vi "test.vi"() -> ()   [LabVIEW 2010, in "AnalysisRaps2.lvclass"]
uses:
  AnalysisRaps2.lvclass
panel:
  out "Array 2":i32[][](array[numeric])
  out "x*y":i32
  out "element 2":i32
  out "element 4":i32
  out "element 3":i32
  out "element":i32
  out "Array":i32[][](array[numeric])
  in  "Numeric":i32
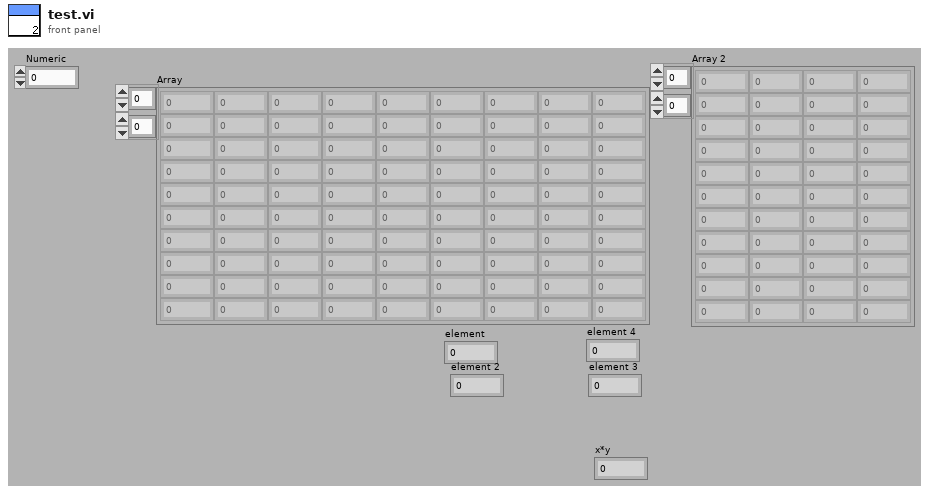
[diagram p1: front panel]
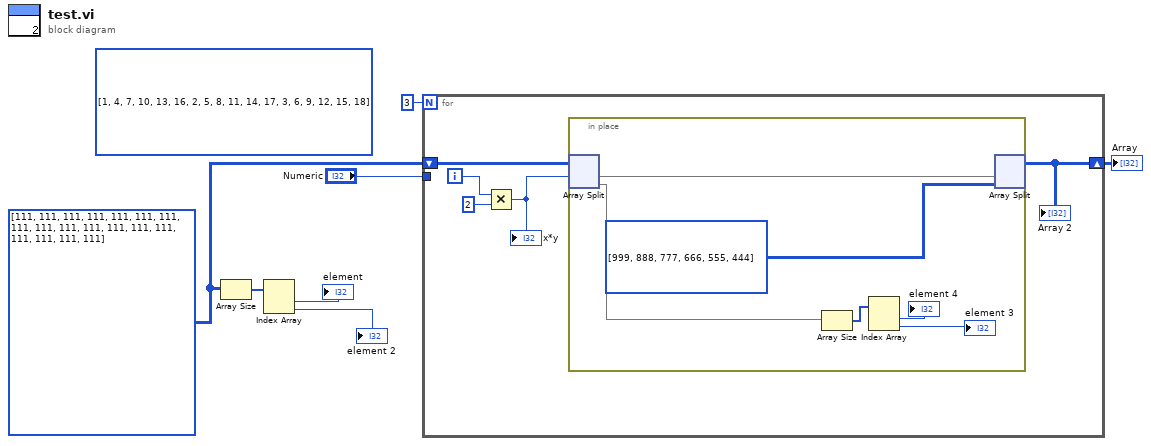
[diagram p0: block diagram]
diagram:
  w5 = i32[][] [[111, 111, 111], [111, 111, 111], [111, 111, 111], [111, 111, 111], [111, 111, 111], [111, 111, 111]]
  (unwired) i32[][] [[1, 4, 7, 10, 13, 16], [2, 5, 8, 11, 14, 17], [3, 6, 9, 12, 15, 18]]
  n1 = Array Size(array=w5) -> (size(s)=w4:i32[])
  n2 = Index Array(array=w4) -> (element #1=→"element":i32, element #2=→"element 2":i32)  [unwired: 2 in]
  n3 = for {
    N: 3 -> [_]
    tunnel: "Numeric" -> [_]
    shift-right: [w11] -> w6
    shift-left: w5 -> [w12]
    i -> [w9]
    n4 = Multiply(x=w9, y=2) -> (x*y=w8:i32)
    "x*y" <- w8
    n5 = in-place {
      n6 = in-place-split #1(w12, w8) -> (w18:i32[][], w13:i32[][])
      n7 = Array Size(array=w13) -> (size(s)=w15:i32[])
      n8 = Index Array(array=w15) -> (element #1=→"element 4":i32, element #2=→"element 3":i32)  [unwired: 2 in]
      n9 = in-place-split #1(w18, i32[][] [[999, 888, 777], [666, 555, 444]]) -> (w11:i32[][])  [unwired: 1 out]
    }
    "Array 2" <- w11
  }
  "Array" <- w6
